vi "Unpack String Value.vi"(11 "StringValueMsg in":refnum<class "StringValueMsg.lvclass">) -> (2 "Value":string, 3 "Name":string)   [LabVIEW 2015, in "ActorAutoRegistration.lvlib" / "StringValueMsg.lvclass"]
uses:
  StringValueMsg.lvclass
  StringValueMsg.lvclass/StringValueMsg.ctl
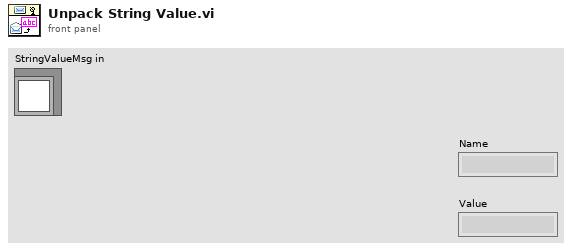
[diagram p1: front panel]
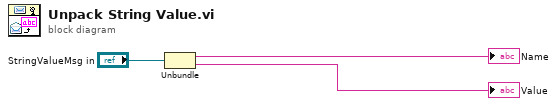
[diagram p0: block diagram]
diagram:
  n1 = Unbundle("StringValueMsg in") -> (→"Name":string, →"Value":string)
